vi "test_serialize_deserialize.vi"   [LabVIEW 2020, in "Signed Quad (I64).lvlib"]
doc: "Version 0.1"
uses:
  <vilib>/ADAS Record/CustomDataTypes/Signed Quad (I64)/Signed Quad (I64).lvlib
  <vilib>/addons/_JKI Toolkits/Caraya/classes/Test/Test.lvclass
  <vilib>/addons/_JKI Toolkits/Caraya/classes/Assert/Assert.lvclass
  <vilib>/ADAS Record/CustomDataTypes/Signed Quad (I64)/Process Data.ctl
  <vilib>/ADAS Record/CustomDataTypes/Signed Quad (I64)/Serialize Data.vi
  <vilib>/ADAS Record/CustomDataTypes/Signed Quad (I64)/Deserialize Data.vi
types:
  T1 = typedef "Signed Quad (I64).lvlib/Process Data.ctl" = cluster{"Time Stamp":timestamp, "Signed Quad (I64)":i64}
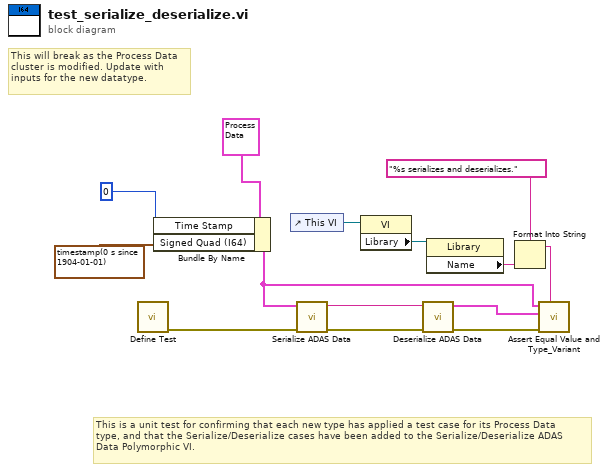
[diagram p0: block diagram]
diagram:
  # "This will break as the Process Data\ncluster is modified. Update with\ninputs for the new datatype."
  # "This is a unit test for confirming that each new type has applied a test case for its Process Data\ntype, and that the Serialize/Deserialize cases have been added to the Serialize/Deserialize ADAS\nData Polymorphic VI."
  n1 = call <vilib>:"Define Test.vi"() -> ("error out"=w9:errorcluster)  [unwired: 11 in]
  n2 = Bundle By Name "Bundle By Name"(cluster=T1 {"Time Stamp"=timestamp(0 s since 1904-01-01), "Signed Quad (I64)"=0} ("Process Data in"), "Time Stamp"=timestamp(0 s since 1904-01-01), "Signed Quad (I64)"=i64 0) -> (w3:T1)
  n3 = control-ref of="This VI"() -> (w14:refnum<vi>)
  n4 = call-poly <vilib>:"Serialize ADAS Data.vi"("error in (no error)"=w9, "Process Data"=w3) -> ("error out"=w8:errorcluster, "Flat Data out"=w7:string)  [unwired: 8 in]
  n5 = property class="VI"(reference=w14) -> ("Library"=w13:refnum<vi>)  [unwired: 1 in, 2 out]
  n6 = call-poly <vilib>:"Deserialize ADAS Data.vi"("error in (no error)"=w8, "Flat Data in"=w7) -> ("error out"=w5:errorcluster, "Process Data out"=w6:T1)  [unwired: 8 in]
  n7 = property class="Library"(reference=w13) -> ("Name"=w11:string)  [unwired: 1 in, 2 out]
  n8 = Format Into String(format string="%s serializes and deserializes.", w11) -> (resulting string=w10:string)  [unwired: 2 in, 1 out]
  n9 = call <vilib>:"Assert Equal Value and Type_Variant.vi"("Label"=w10, "error in (no error)"=w5, "Y"=w6, "X"=w3) -> ()  [unwired: 7 in, 1 out]
